vi "Write Dummy.vi"(8 "error in (no error)":errorcluster, 10 "Dummy":bool, 11 "Instance Handle":T1) -> (0 "error out":errorcluster, 3 "Session Handle":T1)   [LabVIEW 2020, in "singleton.lvclass"]
uses:
  singleton.lvclass
  Typedefs/Instance Handle.ctl
  singleton.lvclass/singleton.ctl
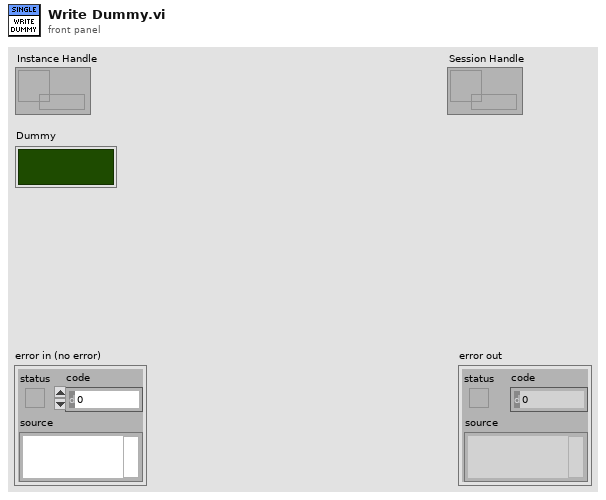
[diagram p1: front panel]
types:
  T1 = typedef "singleton.lvclass/Instance Handle.ctl" = refnum<data-value>
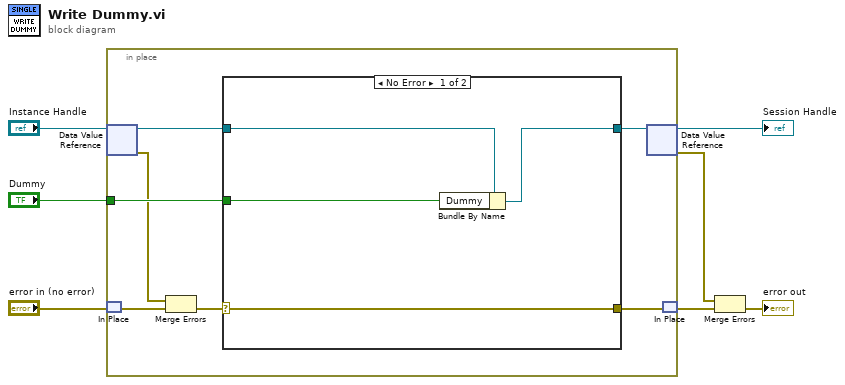
[diagram p0: block diagram]
diagram:
  n1 = in-place {
    in-place-border: "Dummy" -> [w14]
    n2 = in-place-dvr #1("Instance Handle") -> (w9:refnum<class "singleton.lvclass">, w12:errorcluster)
    n3 = in-place-match #2("error in (no error)") -> (w13:errorcluster)
    n4 = Merge Errors(w12, w13) -> (w11:errorcluster)
    n5 = case shown="No Error" w11 {
      selector: w11 -> [w18 w20]
      tunnel: [w18 w20] -> w10
      tunnel: w14 -> [w17 _]
      tunnel: w9 -> [w16 w19]
      tunnel: [w15 w19] -> w8
      frame No Error {
        n6 = Bundle By Name(cluster=w16, "Dummy"=w17) -> (w15:refnum<class "singleton.lvclass">)
      }
      frame Error {
      }
    }
    n7 = in-place-dvr #1(w8) -> (→"Session Handle":T1, w4:errorcluster)
    n8 = in-place-match #2(w10) -> (w5:errorcluster)
  }
  n9 = Merge Errors(w4, w5) -> (→"error out":errorcluster)
